vi "Array2DCartesianToCylindrical.vi"(9 "Y-Vector":dbl[](array[numeric]), 10 "X-Vector":dbl[](array[numeric]), 11 "Cartesian Input Array":dbl[][](graph)) -> (1 "Angle Vector":dbl[](array[numeric]), 2 "RadiusVector":dbl[](array[numeric]), 3 "Cylindrical Output Array":dbl[][](graph))   [LabVIEW 2014]
uses:
  <vilib>/gmath/interp.llb/Create Mesh Grid (2D) (x,y arrays).vi
  <vilib>/gmath/interp.llb/Interpolate 2D (2d X,Y).vi
  <vilib>/gmath/NI_Gmath.lvlib
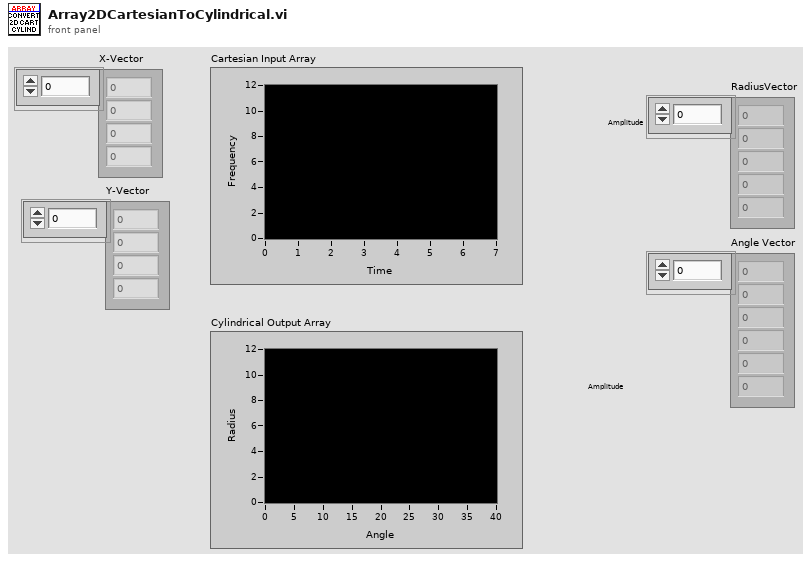
[diagram p1: front panel]
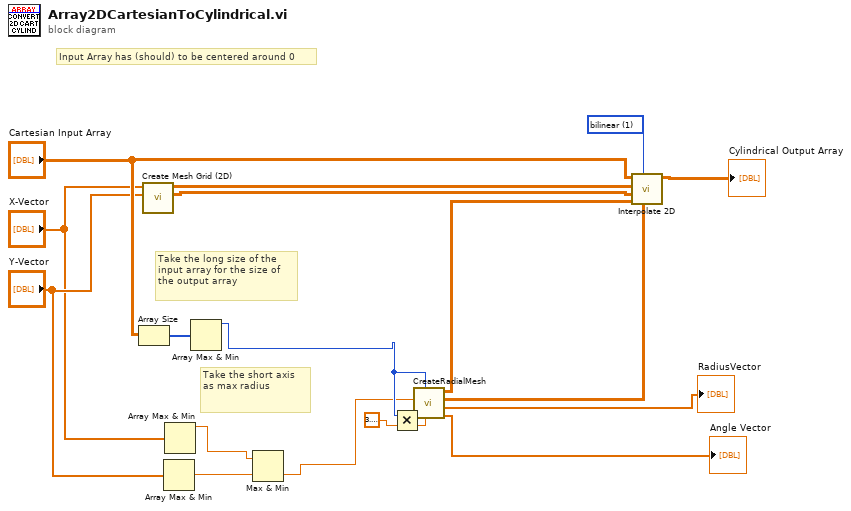
[diagram p0: block diagram]
diagram:
  w13 = 1 items=["nearest", "bilinear", "bicubic", "bicubic spline"] ("method")
  # "Input Array has (should) to be centered around 0"
  # "Take the long size of the input array for the size of the output array"
  # "Take the short axis as max radius"
  n1 = Array Size(array="Cartesian Input Array") -> (size(s)=w9:i32[])
  n2 = call-poly <vilib>:"Create Mesh Grid (2D).vi"("y domain"="Y-Vector", "x domain"="X-Vector") -> ("Y"=w7:dbl[][], "X"=w8:dbl[][])  [unwired: 7 in, 1 out]
  n3 = Array Max & Min(array="Y-Vector") -> (max value=w3:dbl)  [unwired: 3 out]
  n4 = Array Max & Min(array="X-Vector") -> (max value=w4:dbl)  [unwired: 3 out]
  n5 = Array Max & Min(array=w9) -> (max value=w2:i32)  [unwired: 3 out]
  n6 = Max & Min(x=w4, y=w3) -> (min(x,y)=w1:dbl)  [unwired: 1 out]
  n7 = Multiply(x=w2, y=3.141592653589793) -> (x*y=w11:dbl)
  n8 = call "CreateRadialMesh.vi"("AnglePoints"=w11, "RadiusPoints"=w2, "RadiusEnd"=w1) -> ("Angle Vector"=→"Angle Vector":dbl[], "RadiusVector"=→"RadiusVector":dbl[], "RadialMesh Y-Values"=w17:dbl[][], "RadialMesh X-Values"=w12:dbl[][])  [unwired: 3 in]
  n9 = call-poly <vilib>:"Interpolate 2D.vi"("yi"=w17, "method"=w13, "xi"=w12, "Y"=w7, "X"=w8, "Z"="Cartesian Input Array") -> ("zi"=→"Cylindrical Output Array":dbl[][])  [unwired: 2 in, 3 out]
